vi "Read Valve Transfer Line State.vi"(7 "timeout in ms (-1)":i32, 8 "error in (no error)":errorcluster, 11 "Preparation Line in":refnum<class "Preparation Line.lvclass">) -> (0 "error out":errorcluster, 2 "Open?":bool, 3 "Preparation Line out":refnum<class "Preparation Line.lvclass">, 4 "Valve Prep Line StateQ":refnum<queue>)   [LabVIEW 2015, in "cRIO-Carbondioxide.lvlib" / "CO2-Actor.lvlib" / "Preparation Line.lvclass"]
uses:
  Preparation Line.lvclass
  Preparation Line.lvclass/Preparation Line.ctl
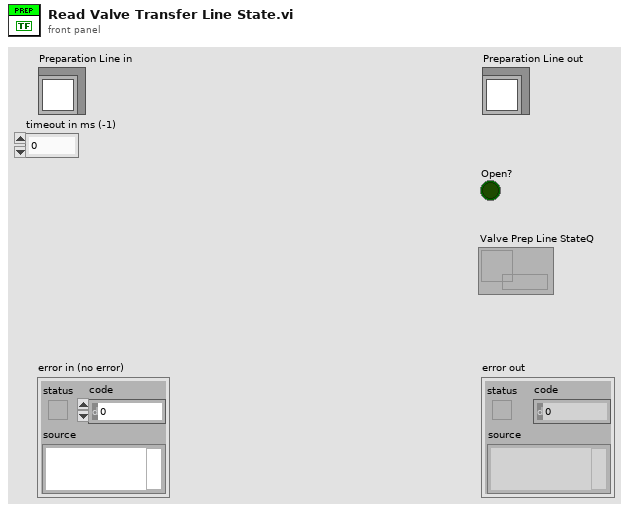
[diagram p1: front panel]
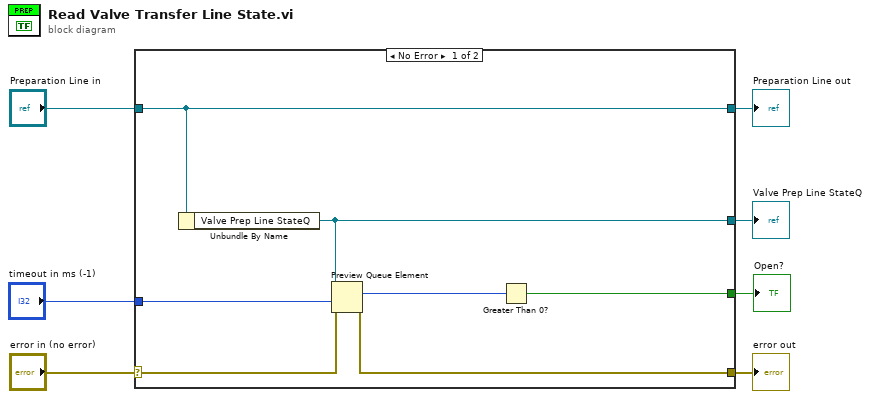
[diagram p0: block diagram]
diagram:
  n1 = case shown="No Error" "error in (no error)" {
    selector: "error in (no error)" -> [w12 w16]
    tunnel: [w11 w16] -> w6
    tunnel: [w13 w15] -> w4
    tunnel: "Preparation Line in" -> [w13 w15]
    tunnel: [w14 _] -> w3
    tunnel: [w9 _] -> w2
    tunnel: "timeout in ms (-1)" -> [w8 _]
    frame No Error {
      n2 = Unbundle By Name(w13) -> ("Valve Prep Line StateQ"=w9:refnum<queue>)
      n3 = Preview Queue Element(queue=w9, timeout in ms (-1)=w8, error in (no error)=w12) -> (element=w10:u16, error out=w11:errorcluster)  [unwired: 2 out]
      n4 = Greater Than 0?(x=w10) -> (x > 0?=w14:bool)
    }
    frame Error {
    }
  }
  "error out" <- w6
  "Preparation Line out" <- w4
  "Open?" <- w3
  "Valve Prep Line StateQ" <- w2
